vi "Text_Get OS Font Names Array.vi"(8 "Error":errorcluster) -> (0 "Error Out":errorcluster, 3 "Font Names Array Out":string[](array[string]))   [LabVIEW 2021]
uses:
  vi.lib/LabVIEW Icon API/lv_icon/lv_icon.lvlib
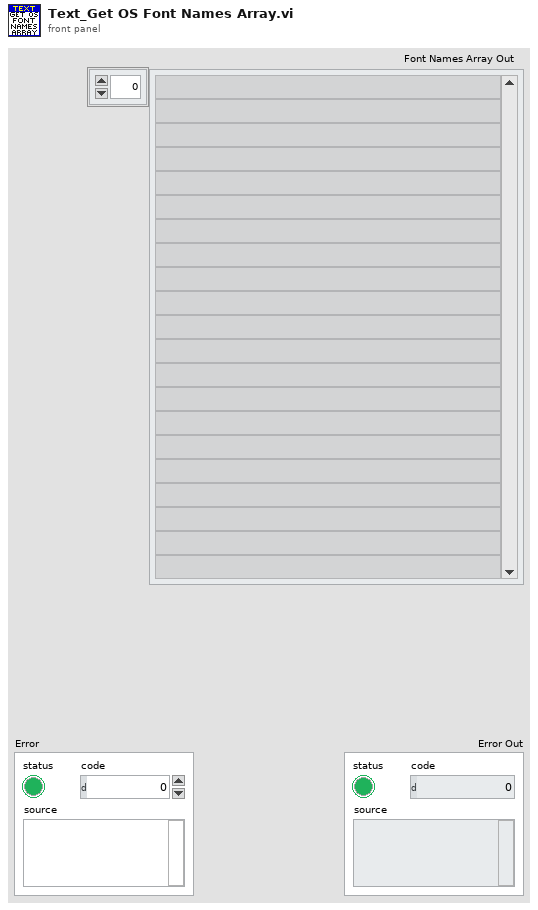
[diagram p1: front panel]
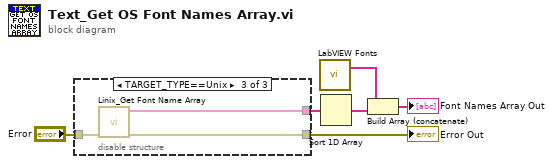
[diagram p0: block diagram]
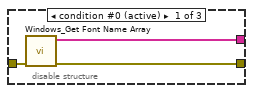
[diagram p2: hidden frame]
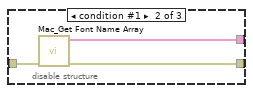
[diagram p3: hidden frame]
diagram:
  n1 = disable-structure shown="TARGET_TYPE==Unix" {
    disable-tunnel: "Error" -> [w9 w12 w15]
    disable-tunnel: [w8 w11 w14] -> w2
    disable-tunnel: [w7 w10 w13] -> w1
    frame condition #0 (active) {
      n2 = call "Windows_Get Font Name Array.vi"("Error"=w9) -> ("Error Out"=w7:errorcluster, "Windows Font Array Out"=w8:string[])  [unwired: 9 in]
    }
    frame condition #1 {
      n3 = call "Mac_Get Font Name Array.vi"("error in (no error)"=w12) -> ("error out"=w10:errorcluster, "Array"=w11:string[])  [unwired: 9 in]
    }
    frame condition #2 {
      n4 = call "Linix_Get Font Name Array.vi"("error in (no error)"=w15) -> ("error out"=w13:errorcluster, "Font Name Array"=w14:string[])  [unwired: 9 in]
    }
  }
  "Error Out" <- w1
  n5 = call "LabVIEW Fonts.vi"() -> ("Additional Fonts"=w5:string[])  [unwired: 1 in, 10 out]
  n6 = Sort 1D Array(array=w2) -> (sorted array=w4:string[])
  n7 = Build Array (concatenate)(w5, w4) -> (→"Font Names Array Out":string[])
